vi "KeyDatabase.vi"() -> ()   [LabVIEW 2023, in "LP_CRC.lvlib"]
uses:
  LP_CRC.lvlib
panel:
  in  "MsgID":string
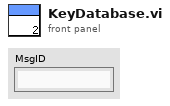
[diagram p1: front panel]
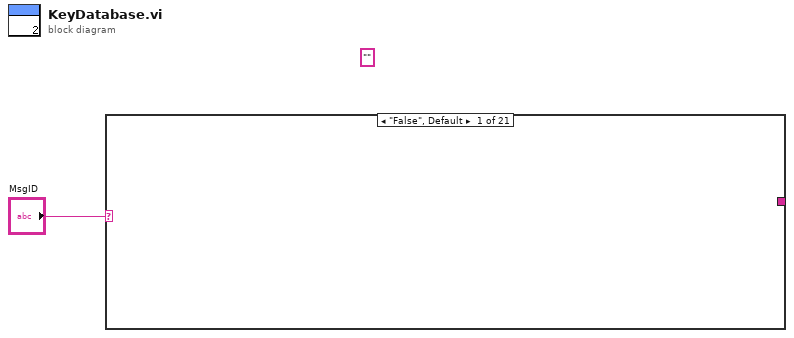
[diagram p0: block diagram]
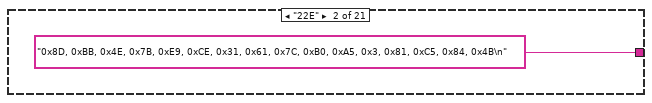
[diagram p2: hidden frame]
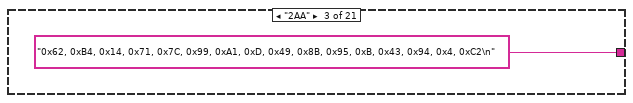
[diagram p3: hidden frame]
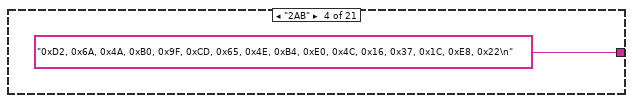
[diagram p4: hidden frame]
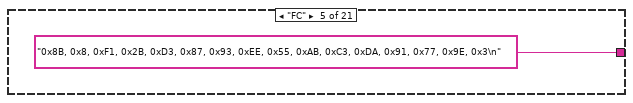
[diagram p5: hidden frame]
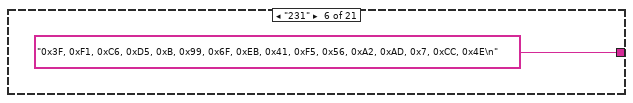
[diagram p6: hidden frame]
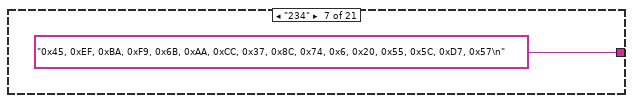
[diagram p7: hidden frame]
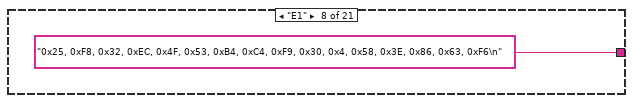
[diagram p8: hidden frame]
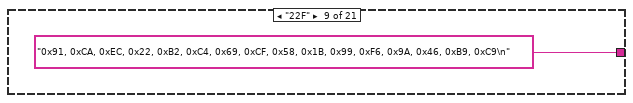
[diagram p9: hidden frame]
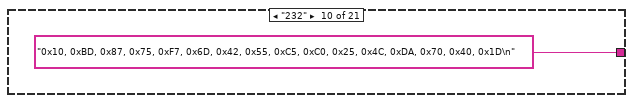
[diagram p10: hidden frame]
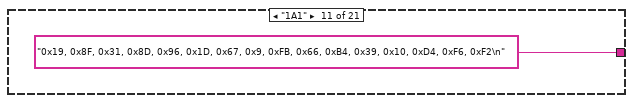
[diagram p11: hidden frame]
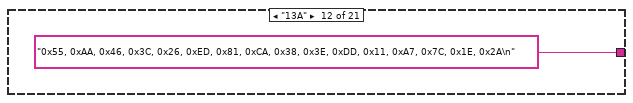
[diagram p12: hidden frame]
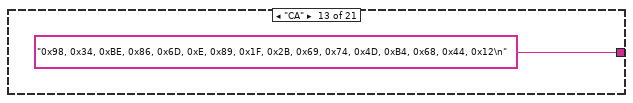
[diagram p13: hidden frame]
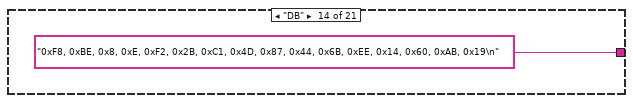
[diagram p14: hidden frame]
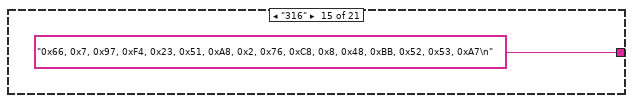
[diagram p15: hidden frame]
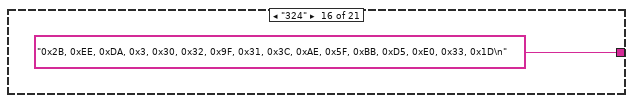
[diagram p16: hidden frame]
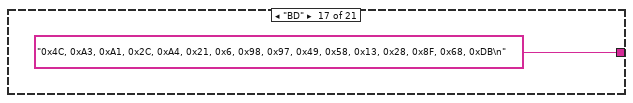
[diagram p17: hidden frame]
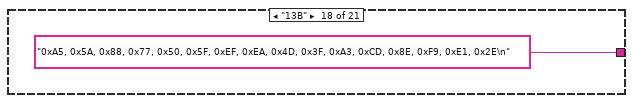
[diagram p18: hidden frame]
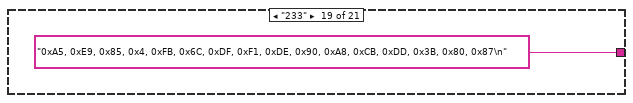
[diagram p19: hidden frame]
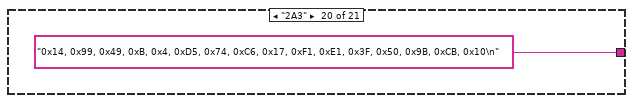
[diagram p20: hidden frame]
diagram:
  (unwired) ""
  n1 = case shown="\"False\", Default" "MsgID" {
    tunnel: [_ "0x8D, 0xBB, 0x4E, 0x7B, 0xE9, 0xCE, 0x31, 0x61, 0x7C, 0xB0, 0xA5, 0x3, 0x81, 0xC5, 0x84, 0x4B\n" "0x62, 0xB4, 0x14, 0x71, 0x7C, 0x99, 0xA1, 0xD, 0x49, 0x8B, 0x95, 0xB, 0x43, 0x94, 0x4, 0xC2\n" "0xD2, 0x6A, 0x4A, 0xB0, 0x9F, 0xCD, 0x65, 0x4E, 0xB4, 0xE0, 0x4C, 0x16, 0x37, 0x1C, 0xE8, 0x22\n" "0x8B, 0x8, 0xF1, 0x2B, 0xD3, 0x87, 0x93, 0xEE, 0x55, 0xAB, 0xC3, 0xDA, 0x91, 0x77, 0x9E, 0x3\n" "0x3F, 0xF1, 0xC6, 0xD5, 0xB, 0x99, 0x6F, 0xEB, 0x41, 0xF5, 0x56, 0xA2, 0xAD, 0x7, 0xCC, 0x4E\n" "0x45, 0xEF, 0xBA, 0xF9, 0x6B, 0xAA, 0xCC, 0x37, 0x8C, 0x74, 0x6, 0x20, 0x55, 0x5C, 0xD7, 0x57\n" "0x25, 0xF8, 0x32, 0xEC, 0x4F, 0x53, 0xB4, 0xC4, 0xF9, 0x30, 0x4, 0x58, 0x3E, 0x86, 0x63, 0xF6\n" "0x91, 0xCA, 0xEC, 0x22, 0xB2, 0xC4, 0x69, 0xCF, 0x58, 0x1B, 0x99, 0xF6, 0x9A, 0x46, 0xB9, 0xC9\n" "0x10, 0xBD, 0x87, 0x75, 0xF7, 0x6D, 0x42, 0x55, 0xC5, 0xC0, 0x25, 0x4C, 0xDA, 0x70, 0x40, 0x1D\n" "0x19, 0x8F, 0x31, 0x8D, 0x96, 0x1D, 0x67, 0x9, 0xFB, 0x66, 0xB4, 0x39, 0x10, 0xD4, 0xF6, 0xF2\n" "0x55, 0xAA, 0x46, 0x3C, 0x26, 0xED, 0x81, 0xCA, 0x38, 0x3E, 0xDD, 0x11, 0xA7, 0x7C, 0x1E, 0x2A\n" "0x98, 0x34, 0xBE, 0x86, 0x6D, 0xE, 0x89, 0x1F, 0x2B, 0x69, 0x74, 0x4D, 0xB4, 0x68, 0x44, 0x12\n" "0xF8, 0xBE, 0x8, 0xE, 0xF2, 0x2B, 0xC1, 0x4D, 0x87, 0x44, 0x6B, 0xEE, 0x14, 0x60, 0xAB, 0x19\n" "0x66, 0x7, 0x97, 0xF4, 0x23, 0x51, 0xA8, 0x2, 0x76, 0xC8, 0x8, 0x48, 0xBB, 0x52, 0x53, 0xA7\n" "0x2B, 0xEE, 0xDA, 0x3, 0x30, 0x32, 0x9F, 0x31, 0x3C, 0xAE, 0x5F, 0xBB, 0xD5, 0xE0, 0x33, 0x1D\n" "0x4C, 0xA3, 0xA1, 0x2C, 0xA4, 0x21, 0x6, 0x98, 0x97, 0x49, 0x58, 0x13, 0x28, 0x8F, 0x68, 0xDB\n" "0xA5, 0x5A, 0x88, 0x77, 0x50, 0x5F, 0xEF, 0xEA, 0x4D, 0x3F, 0xA3, 0xCD, 0x8E, 0xF9, 0xE1, 0x2E\n" "0xA5, 0xE9, 0x85, 0x4, 0xFB, 0x6C, 0xDF, 0xF1, 0xDE, 0x90, 0xA8, 0xCB, 0xDD, 0x3B, 0x80, 0x87\n" "0x14, 0x99, 0x49, 0xB, 0x4, 0xD5, 0x74, 0xC6, 0x17, 0xF1, 0xE1, 0x3F, 0x50, 0x9B, 0xCB, 0x10\n" "0xC5, 0x9E, 0x5D, 0xA1, 0xAC, 0x96, 0x1B, 0x21, 0x82, 0xEE, 0xF9, 0x97, 0xB1, 0xCB, 0xB6, 0x13\n"] -> _
    frame "False", Default {
    }
    frame "22E" {
    }
    frame "2AA" {
    }
    frame "2AB" {
    }
    frame "FC" {
    }
    frame "231" {
    }
    frame "234" {
    }
    frame "E1" {
    }
    frame "22F" {
    }
    frame "232" {
    }
    frame "1A1" {
    }
    frame "13A" {
    }
    frame "CA" {
    }
    frame "DB" {
    }
    frame "316" {
    }
    frame "324" {
    }
    frame "BD" {
    }
    frame "13B" {
    }
    frame "233" {
    }
    frame "2A3" {
    }
    frame "228" {
    }
  }
